vi "Do Request.vi"(7 "Processing In":refnum<class "Processing.lvclass">, 11 "TimerStatusController in":refnum<class "TimerStatusController.lvclass">) -> (0 "error out":errorcluster, 5 "Processing":refnum<class "Processing.lvclass">)   [LabVIEW 2020, in "Timer Demo.lvlib" / "TimerStatusController.lvclass"]
uses:
  TimerStatusController.lvclass
  <vilib>/IlluminatedG/IG HTTP Server/HTTP Server/Processing/Processing.lvclass
  Timer Status Response.ctl
  Timer Status Request.ctl
  TimerStatusController.lvclass/TimerStatusController.ctl
  <vilib>/IlluminatedG/IG HTTP Server/HTTP Server/Processing/Processing.lvclass/Processing.ctl
  Timer Demo.lvlib
  <vilib>/IlluminatedG/IG HTTP Utils/HTTP Utils/Response/Response.lvclass
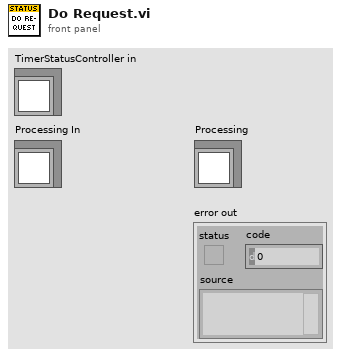
[diagram p1: front panel]
types:
  T1 = typedef "Timer Demo.lvlib/Timer Status Request.ctl" = cluster{"Response":refnum<notifier>}
  T2 = typedef "Timer Demo.lvlib/Timer Status Response.ctl" = cluster{"Elapsed":dbl, "Running":bool}
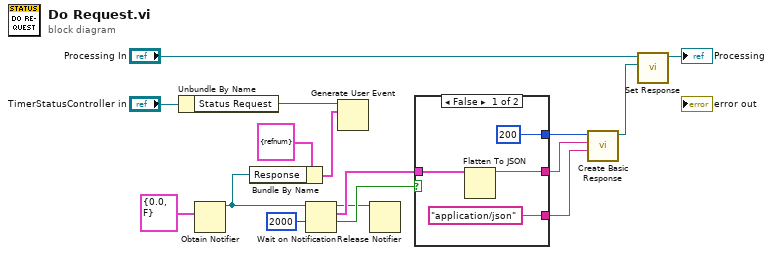
[diagram p0: block diagram]
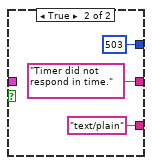
[diagram p2: hidden frame]
diagram:
  n1 = Unbundle By Name("TimerStatusController in") -> ("Status Request"=w14:refnum<user-event>)
  n2 = Obtain Notifier(notification data type=T2 {"Elapsed"=0.0, "Running"=FALSE} ("Timer Status Response")) -> (notifier out=w11:refnum<notifier>)  [unwired: 3 in, 2 out]
  n3 = Bundle By Name(cluster=T1 {"Response"=refnum} ("event data"), "Response"=w11) -> (w12:T1)
  n4 = Wait on Notification(notifier=w11, timeout in ms (-1)=2000) -> (notifier out=w7:refnum<notifier>, notification=w9:T2, timed out?=w8:bool)  [unwired: 2 in, 1 out]
  n5 = Generate User Event(user event=w14, event data cluster=w12) -> ()  [unwired: 2 in, 2 out]
  n6 = Release Notifier(notifier=w7) -> ()  [unwired: 2 in, 3 out]
  n7 = case shown="False" w8 {
    tunnel: w9 -> [w20 _]
    tunnel: [u16 200 ("Status Code") u16 503 ("Status Code")] -> w3
    tunnel: [w18 "Timer did not respond in time." ("JSON string")] -> w2
    tunnel: ["application/json" ("Content-Type (text/plain)") "text/plain" ("Content-Type (text/plain)")] -> w1
    frame False {
      n8 = Flatten To JSON(anything=w20) -> (JSON string=w18:string)  [unwired: 2 in, 1 out]
    }
    frame True {
    }
  }
  n9 = call <vilib>:"Create Basic Response.vi"("Content-Type (text/plain)"=w1, "Payload"=w2, "Status Code"=w3) -> ("Response out"=w4:refnum<class "Response.lvclass">)  [unwired: 7 in, 1 out]
  n10 = call <vilib>:"Set Response.vi"("Response"=w4, "Processing in"="Processing In") -> ("Processing out"=→"Processing":refnum<class "Processing.lvclass">)  [unwired: 9 in]
